vi "Region-det-init-queue.vi"(8 "error in (no error)":errorcluster) -> (0 "error out":errorcluster, 3 "Queues":T1)   [LabVIEW 2016]
uses:
  Sched_queues.ctl
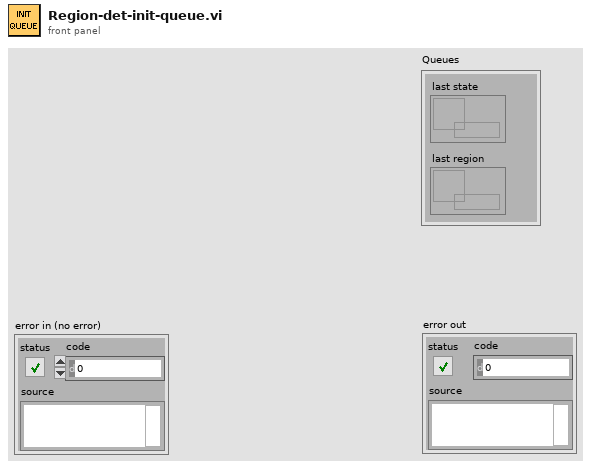
[diagram p1: front panel]
types:
  T1 = typedef "Sched_queues.ctl" = cluster{"last region":refnum<queue>, "last state":refnum<queue>}
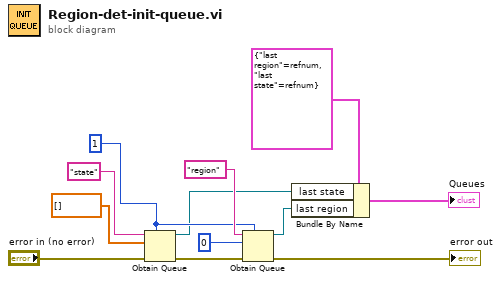
[diagram p0: block diagram]
diagram:
  w9 = 1 ("max queue size (-1, unlimited)")
  n1 = Obtain Queue(max queue size (-1, unlimited)=w9, name (unnamed)="state", element data type=dbl[] [], error in (no error)="error in (no error)") -> (queue out=w2:refnum<queue>, error out=w6:errorcluster)  [unwired: 1 in, 1 out]
  n2 = Obtain Queue(max queue size (-1, unlimited)=w9, name (unnamed)="region", element data type=0, error in (no error)=w6) -> (queue out=w1:refnum<queue>, error out=→"error out":errorcluster)  [unwired: 1 in, 1 out]
  n3 = Bundle By Name(cluster=T1 {"last region"=refnum, "last state"=refnum} ("Queues 2"), "last state"=w2, "last region"=w1) -> (→"Queues":T1)
